vi "Actor Core.vi"(8 "error in":errorcluster, 11 "Orca-Flash 4.0 V2 in":refnum<class "Hamamatsu Camera.lvclass">) -> (0 "error out":errorcluster, 3 "Actor out":refnum<class "Actor.lvclass">)   [LabVIEW 2018, in "Hamamatsu Camera.lvlib" / "Hamamatsu Camera.lvclass"]
doc: "(<B>Filename</B>: Actor Framework.lvlib:Actor.lvclass:Actor Core.vi)\n\nReceives messages to the actor, reacts to them, and initiates any error handling that may shut the actor down.\n\nDescendant classes may override this VI to append parallel tasks for the actor to complete while it handles messages. Overrides use the Call Parent Method node."
uses:
  Hamamatsu Camera.lvclass
  C:/Program Files/National Instruments/LabVIEW 2018/vi.lib/ActorFramework/Actor/Actor.lvclass
  <vilib>/ActorFramework/Actor/Actor.lvclass
  <vilib>/ActorFramework/Actor/Actor.lvclass/Actor.ctl
  <vilib>/ActorFramework/Message Enqueuer/Message Enqueuer.lvclass/Message Enqueuer.ctl
  <vilib>/ActorFramework/Message Enqueuer/Message Priority.ctl
  <vilib>/ActorFramework/Message Enqueuer/Init from Existing Queue.vi
  <vilib>/ActorFramework/Message Enqueuer/Enqueue.vi
  Hamamatsu Camera Messages/Get Most Recent Frame (if active) Msg/Get Most Recent Frame (if active) Msg.lvclass
  C:/Program Files/National Instruments/LabVIEW 2018/vi.lib/ActorFramework/Message/Message.lvclass
  Resources/GLOBAL/GLOBAL Time-critical.vi
  <vilib>/ActorFramework/Message Priority Queue/Priority Enqueue.vi
  Camera/Camera.lvclass
  <vilib>/ActorFramework/Message Enqueuer/Message Enqueuer.lvclass
panel:
  in  "Stop Button":bool
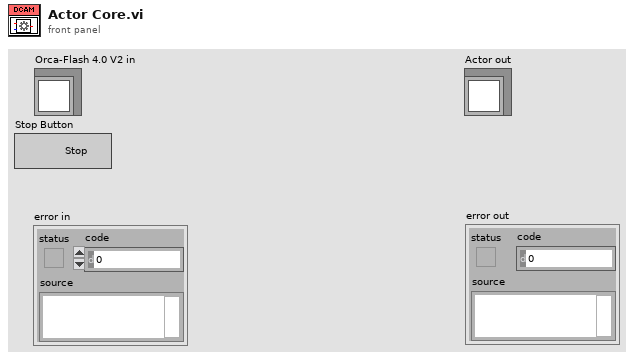
[diagram p1: front panel]
types:
  T1 = typedef "Actor Framework.lvlib/Message Enqueuer.lvclass/Message Priority.ctl" = enum16{"Low", "Normal", "High"}
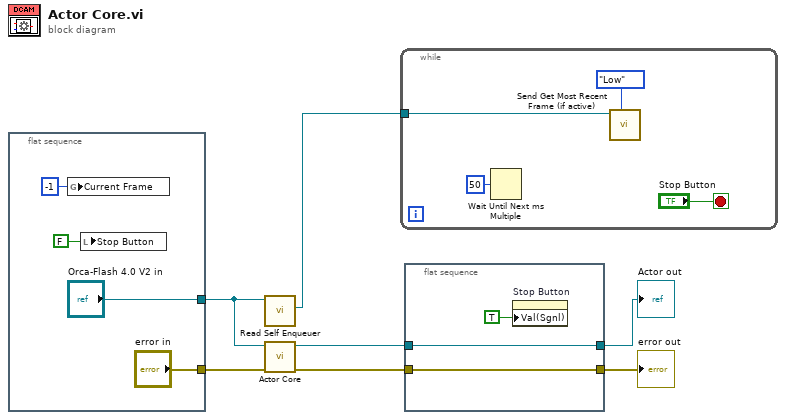
[diagram p0: block diagram]
diagram:
  n1 = flat-sequence {
    tunnel: ["error in"] -> w7
    tunnel: ["Orca-Flash 4.0 V2 in"] -> w1
    frame #0 {
      n2 = global write "GLOBAL Time-critical.vi" "Current Frame"(-1 ("Current Frame")) -> ()
      n3 = local write "Stop Button"(FALSE ("Stop Button")) -> ()
    }
  }
  n4 = call <vilib>:"Read Self Enqueuer.vi"("Actor"=w1) -> ("Self Enqueuer"=w2:refnum<class "Message Enqueuer.lvclass">)  [unwired: 10 in]
  n5 = call-parent "Actor Core.vi"("error in"=w7, "Device in"=w1) -> ("error out"=w4:errorcluster, "Actor out"=w6:refnum<class "Actor.lvclass">)  [unwired: 8 in]
  n6 = while {
    tunnel: w2 -> [w14]
    stop <- "Stop Button" stop-if-true
    n7 = Wait Until Next ms Multiple(millisecond multiple=u32 50) -> ()  [unwired: 1 out]
    n8 = call "Send Get Most Recent Frame (if active).vi"("Message Priority (Normal)"=Message_Priority."Low", "Message Enqueuer"=w14) -> ()  [unwired: 8 in, 2 out]
  }
  n9 = flat-sequence {
    tunnel: w6 -> [w17]
    tunnel: [w17] -> w5
    tunnel: w4 -> [w16]
    tunnel: [w16] -> w3
    frame #0 {
      n10 = property on="Stop Button" class="Bool (strict)"("Val(Sgnl)"=TRUE) -> ()  [unwired: 2 in, 2 out]
    }
  }
  "error out" <- w3
  "Actor out" <- w5
